vi "Dev1_timing_source.vi"() -> (3 "timing source out":string)   [LabVIEW 2016]
uses:
  <vilib>/DAQmx/create/channels.llb/DAQmx Create Channel (AI-Voltage-Basic).vi
  <vilib>/DAQmx/configure/timing.llb/DAQmx Timing (Sample Clock).vi
  <vilib>/DAQmx/create/timing.llb/DAQmx Create Timing Source (Control Loop From Task).vi
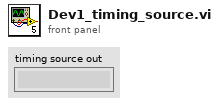
[diagram p1: front panel]
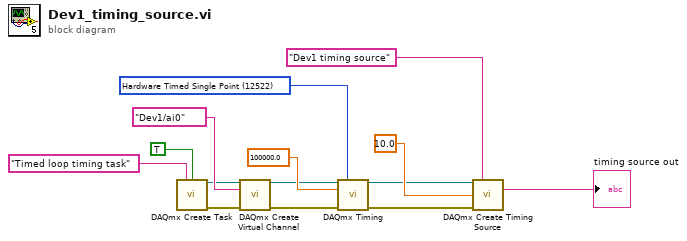
[diagram p0: block diagram]
diagram:
  w6 = 12522 items=["Finite Samples"=10178, "Continuous Samples"=10123, "Hardware Timed Single Point"=12522] ("sample mode")
  n1 = call <vilib>:"DAQmx Create Task.vi"("new task name"="Timed loop timing task", "auto cleanup"=TRUE) -> ("task out"=w1:refnum<k21>, "error out"=w2:errorcluster)  [unwired: 12 in]
  n2 = call-poly <vilib>:"DAQmx Create Virtual Channel.vi"("task in"=w1, "physical channels"=tag "Dev1/ai0", "error in"=w2) -> ("task out"=w4:refnum<k21>, "error out"=w5:errorcluster)  [unwired: 11 in]
  n3 = call-poly <vilib>:"DAQmx Timing.vi"("task/channels in"=w4, "sample mode"=w6, "rate"=100000.0, "error in"=w5) -> ("task out"=w7:refnum<k21>, "error out"=w8:errorcluster)  [unwired: 10 in]
  n4 = call-poly <vilib>:"DAQmx Create Timing Source.vi"("task/channels in"=w7, "timing source name"="Dev1 timing source", "sleep time (us)"=10.0, "error in"=w8) -> ("timing source out"=→"timing source out":string)  [unwired: 9 in, 2 out]
